vi "GSE 350 Extract Negative Value.vi"(8 "Error In":errorcluster, 9 "Regular Expression Search":string, 10 "Full String":string, 11 "Expression With Negative Search":string) -> (0 "Error Out":errorcluster, 1 "Negative Number?":bool, 2 "Found Match":bool, 3 "Output Match":string)   [LabVIEW 2018]
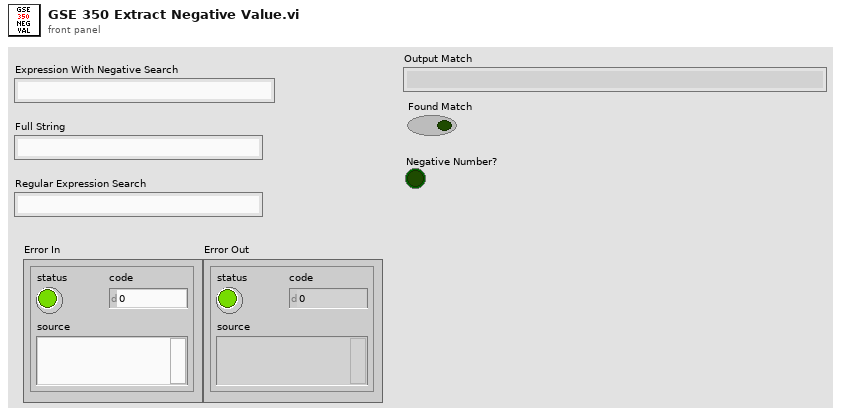
[diagram p1: front panel]
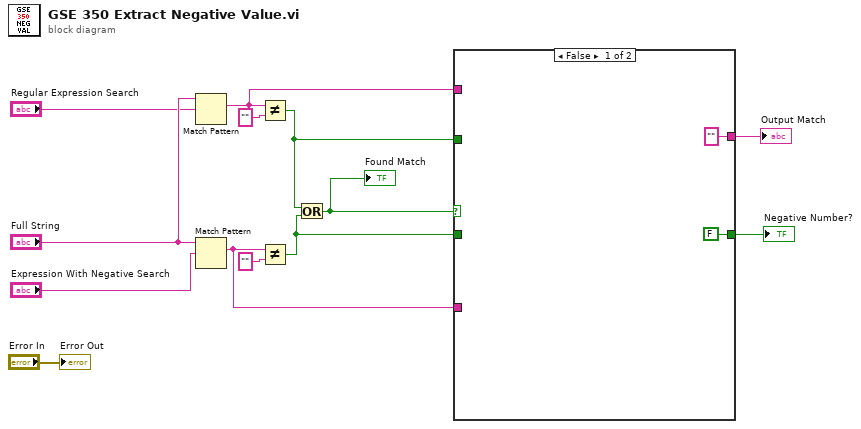
[diagram p0: block diagram]
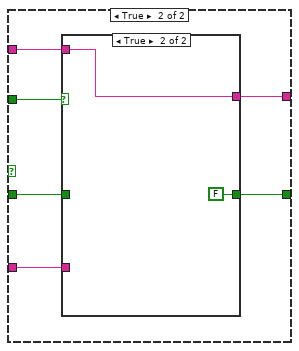
[diagram p2: hidden frame]
diagram:
  n1 = Match Pattern(string="Full String", regular expression="Regular Expression Search") -> (match substring=w6:string)  [unwired: 1 in, 3 out]
  n2 = Match Pattern(string="Full String", regular expression="Expression With Negative Search") -> (match substring=w3:string)  [unwired: 1 in, 3 out]
  n3 = Not Equal?(x=w6, y="") -> (x != y?=w5:bool)
  n4 = Not Equal?(x=w3, y="") -> (x != y?=w2:bool)
  n5 = Or(x=w5, y=w2) -> (x .or. y?=w7:bool)
  "Found Match" <- w7
  n6 = case shown="False" w7 {
    tunnel: w6 -> [_ w20]
    tunnel: w5 -> [_ w21]
    tunnel: ["" ("Full String") w19] -> w4
    tunnel: w3 -> [_ w18]
    tunnel: w2 -> [_ w17]
    tunnel: [FALSE w16] -> w1
    frame False {
    }
    frame True {
      n7 = case shown="True" w21 {
        tunnel: w20 -> [_ w25]
        tunnel: [w23 w25] -> w19
        tunnel: w18 -> [w23 _]
        tunnel: w17 -> [w22 _]
        tunnel: [w22 FALSE] -> w16
        frame False {
        }
        frame True {
        }
      }
    }
  }
  "Output Match" <- w4
  "Negative Number?" <- w1
  "Error Out" <- "Error In"
